vi "Format Port ID.vi"(11 "port":i32) -> (3 "formatted port ID":string)   [LabVIEW 2014, in "GraphViz Mapping Visualizer.lvlib"]
uses:
  GraphViz Mapping Visualizer.lvlib
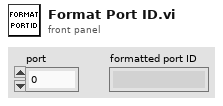
[diagram p1: front panel]
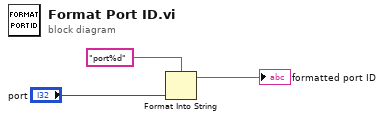
[diagram p0: block diagram]
diagram:
  n1 = Format Into String(format string="port%d", "port") -> (resulting string=→"formatted port ID":string)  [unwired: 2 in, 1 out]
